vi "Throw Async Handler Error.vi"(8 "error in (no error)":errorcluster, 10 "Error":errorcluster, 11 "Mock Async Handler Process in":refnum<class "Mock Async Handler Process.lvclass">) -> (0 "error out":errorcluster, 3 "Mock Async Handler Process out":refnum<class "Mock Async Handler Process.lvclass">)   [LabVIEW 2020, in "Mock Async Handler Process.lvclass"]
uses:
  Mock Async Handler Process.lvclass
  C:/Git/astemes-triarc-framework/source/Framework/Process/Process.lvclass
  source/Framework/Process/Process.lvclass/Process.ctl
  source/Framework/Process/Public/Lifecycle/Get Lifecycle State.vi
  source/Framework/Process/Private/SubVIs/Handle Debug Data.vi
  <vilib>/Utility/error.llb/Clear Errors.vi
  source/Framework/Logging/Log Debug.vi
  <vilib>/AdvancedString/1D String Array to Delimited String.vi
  <vilib>/Utility/High Resolution Relative Seconds.vi
  <vilib>/Utility/error.llb/Error Cluster From Error Code.vi
  source/Framework/Process/Public/Read Name.vi
  source/Framework/Process/Process.lvclass
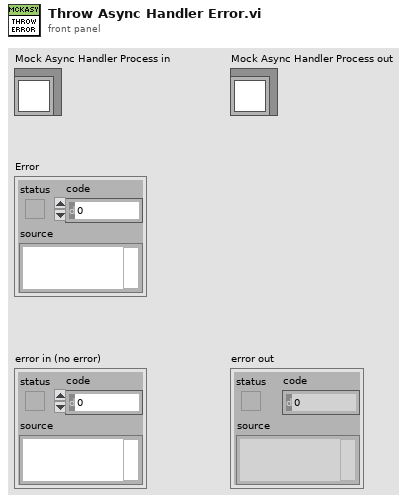
[diagram p1: front panel]
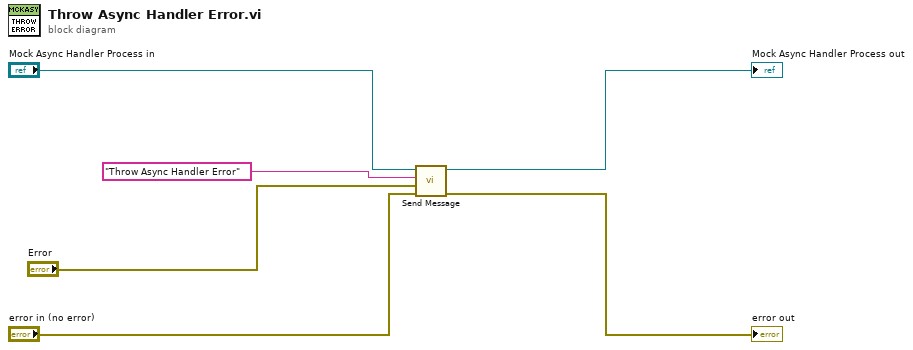
[diagram p0: block diagram]
diagram:
  n1 = call "Send Message.vi"("error in (no error)"="error in (no error)", "Message Data"="Error", "Message"="Throw Async Handler Error", "Process In"="Mock Async Handler Process in") -> ("error out"=→"error out":errorcluster, "Process Out"=→"Mock Async Handler Process out":refnum<class "Mock Async Handler Process.lvclass">)  [unwired: 6 in]
